vi "Read Analog Output Data.vi"(8 "error in (no error)":errorcluster, 10 "Output (0:Sample Heater)":u16(ring) items=["Sample Heater", "Warm-up Heater (Output 1)"], 11 "VISA resource name":refnum<visa-resource-name>) -> (0 "error out":errorcluster, 2 "Analog Output":dbl min=-100.0 max=100.0 step=1e-05 format="%^.5e", 3 "VISA resource name out":refnum<visa-resource-name>)   [LabVIEW 2015, in "Lake Shore 372.lvlib"]
doc: "Returns the percentage of output of the analog output."
uses:
  <instrlib>/Lake Shore 372/Lake Shore 372.lvlib
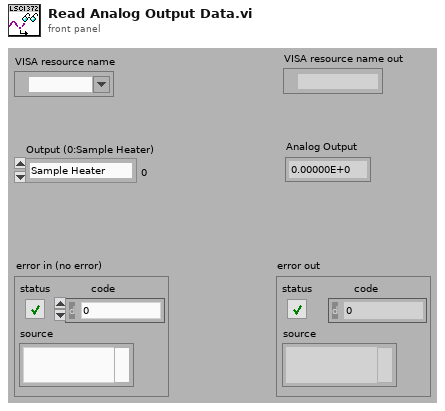
[diagram p1: front panel]
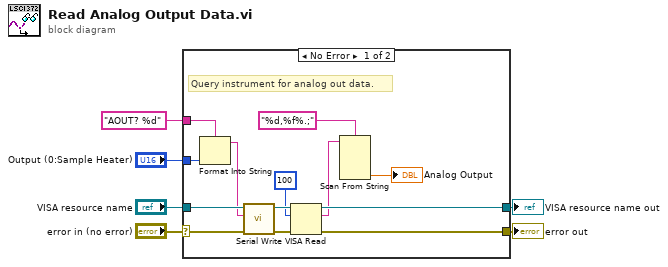
[diagram p0: block diagram]
diagram:
  n1 = case shown="No Error" "error in (no error)" {
    selector: "error in (no error)" -> [w8 w20]
    tunnel: "VISA resource name" -> [w16 w21]
    tunnel: [w15 w21] -> w5
    tunnel: [w14 w20] -> w4
    tunnel: "AOUT? %d" ("format string") -> [w13 _]
    tunnel: "Output (0:Sample Heater)" -> [w12 _]
    frame No Error {
      # "Query instrument for analog out data."
      n2 = Format Into String(format string=w13, w12) -> (resulting string=w11:string)  [unwired: 2 in, 1 out]
      n3 = call <instrlib>:"Serial Write.vi"("error in (no error)"=w8, "Write Buffer (\"\")"=w11, "VISA resource name"=w16) -> ("error out"=w18:errorcluster, "VISA resource name out"=w19:refnum<visa-resource-name>)  [unwired: 6 in, 1 out]
      n4 = VISA Read(VISA resource name=w19, byte count=100, error in (no error)=w18) -> (VISA resource name out=w15:refnum<visa-resource-name>, read buffer=w7:string, error out=w14:errorcluster)  [unwired: 1 out]
      n5 = Scan From String(format string="%d,%f%.;", input string=w7) -> (output 2=→"Analog Output":dbl)  [unwired: 5 in, 3 out]
    }
    frame Error {
    }
  }
  "error out" <- w4
  "VISA resource name out" <- w5
